vi "PID.vi"() -> ()   [LabVIEW 2014]
panel:
  in  "Stack Level":dbl
  in  "Encoder Output":dbl[](array[numeric])
  in  "Joystick Input":dbl
  out "Motor Output":dbl[](array[numeric])
  in  "Motor Input":dbl[](array[numeric])
  in  "Base Level PID constants":dbl[](array[numeric])
  # "Proportional Constant"
  # "Integral Constant"
  # "Derivative Constant"
  # "Feed Forward Constant"
  # "Front Left"
  # "Front Left"
  # "Rear Left"
  # "Rear Left"
  # "Front Right"
  # "Front Right"
  # "Rear Right"
  # "Rear Right"
  # "Front Left"
  # "Rear Left"
  # "Front Right"
  # "Rear Right"
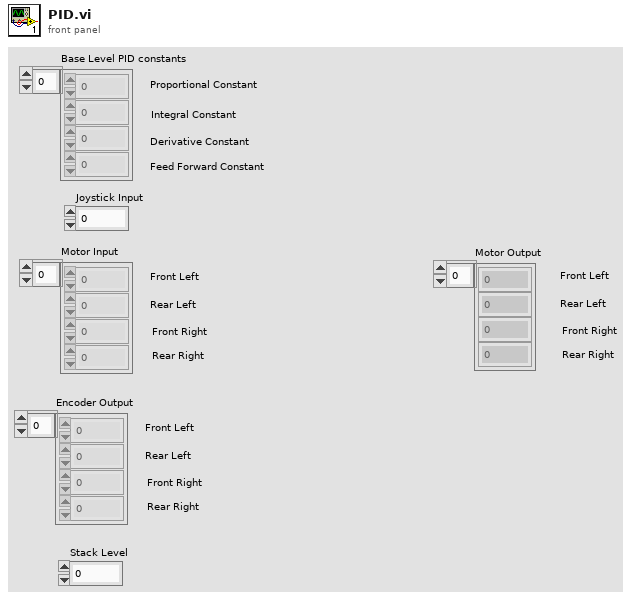
[diagram p1: front panel]
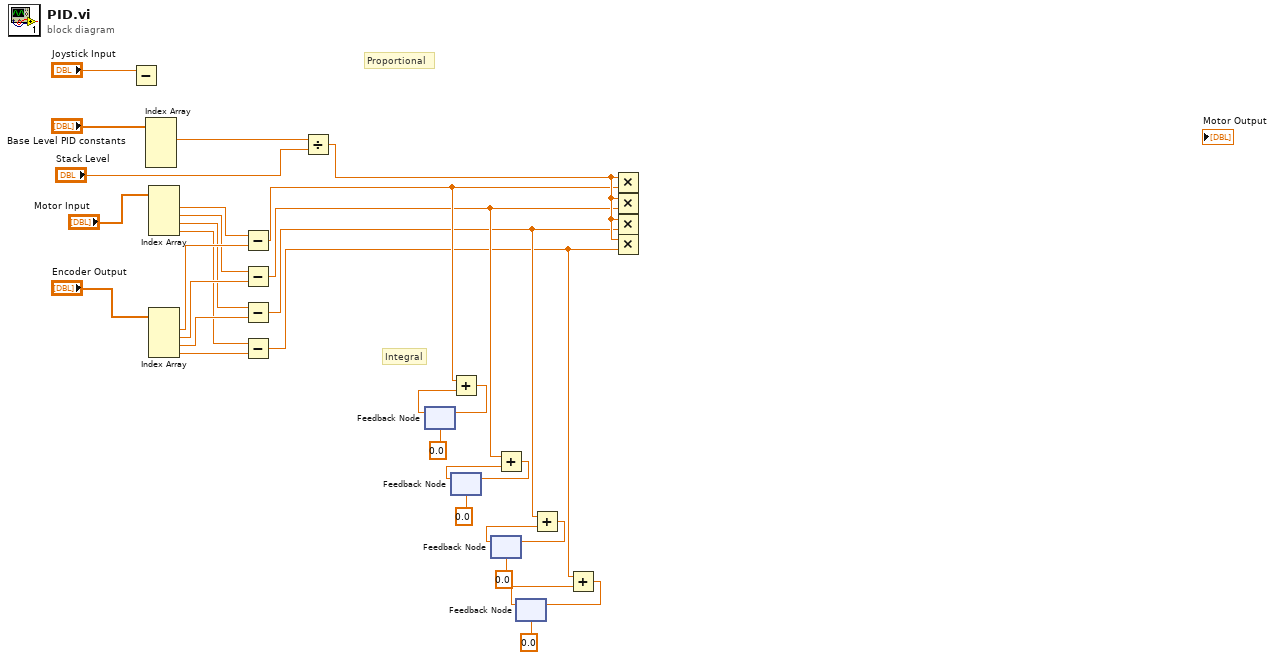
[diagram p0: block diagram]
diagram:
  # "Integral"
  # "Proportional"
  n1 = Subtract(x="Joystick Input") -> ()  [unwired: 1 in, 1 out]
  n2 = Index Array(array="Base Level PID constants") -> (element #1=w14:dbl)  [unwired: 4 in, 3 out]
  n3 = Index Array(array="Motor Input") -> (element #1=w28:dbl, element #2=w20:dbl, element #3=w25:dbl, element #4=w23:dbl)  [unwired: 4 in]
  n4 = Index Array(array="Encoder Output") -> (element #1=w27:dbl, element #2=w26:dbl, element #3=w24:dbl, element #4=w22:dbl)  [unwired: 4 in]
  n5 = Subtract(x=w28, y=w27) -> (x-y=w12:dbl)
  n6 = Subtract(x=w20, y=w26) -> (x-y=w9:dbl)
  n7 = Subtract(x=w25, y=w24) -> (x-y=w6:dbl)
  n8 = Subtract(x=w23, y=w22) -> (x-y=w2:dbl)
  n9 = Divide(x=w14, y="Stack Level") -> (x/y=w13:dbl)
  n10 = feedback #1(0.0) -> (w11:dbl)
  n11 = Add(x=w12, y=w11) -> (x+y=w10:dbl)
  n12 = feedback-in #1(w10) -> ()
  n13 = feedback #2(0.0) -> (w8:dbl)
  n14 = feedback #3(0.0) -> (w4:dbl)
  n15 = Add(x=w9, y=w8) -> (x+y=w7:dbl)
  n16 = feedback-in #2(w7) -> ()
  n17 = feedback #4(0.0) -> (w3:dbl)
  n18 = Add(x=w6, y=w4) -> (x+y=w5:dbl)
  n19 = feedback-in #3(w5) -> ()
  n20 = Add(x=w2, y=w3) -> (x+y=w1:dbl)
  n21 = feedback-in #4(w1) -> ()
  n22 = Multiply(x=w13, y=w12) -> ()  [unwired: 1 out]
  n23 = Multiply(x=w13, y=w9) -> ()  [unwired: 1 out]
  n24 = Multiply(x=w13, y=w6) -> ()  [unwired: 1 out]
  n25 = Multiply(x=w13, y=w2) -> ()  [unwired: 1 out]
